vi "Shoot into low goal.vi"(6 "navX Device":T1 {"Interface"."Update Rate (4Hz-60Hz)" min=4 max=60 step=1}, 8 "Enum":enum16{"5", "4", "3", "2", "1"}(ring), 9 "SonarMB1010AnalogDevRef":T11 {"Average Bits" max=15}, 10 "MotorControlDevRef":T4, 11 "RobotDriveDevRef":T3) -> ()   [LabVIEW 2015]
uses:
  <vilib>/Rock Robotics/WPI/MotorControl/WPI_MotorControlDeviceRef.ctl
  <vilib>/Rock Robotics/WPI/MotorControl/WPI_MotorControlType.ctl
  <vilib>/Rock Robotics/SystemInterfaces/DIO/FPGA_DIOPWMChannel.ctl
  <vilib>/Rock Robotics/WPI/PWM/WPI_PWMDeadband.ctl
  <vilib>/Rock Robotics/WPI/CAN/Jaguar/SubVIs/WPI_CANJaguar_ControlMode.ctl
  <vilib>/Rock Robotics/WPI/CAN/TalonSRX/WPI_CANTalonSRX_APIControlMode.ctl
  <vilib>/Rock Robotics/WPI/Ultrasonic/WPI_SonarMB1010AnalogDeviceRef.ctl
  <vilib>/Rock Robotics/WPI/AnalogChannel/WPI_AnalogChannelDevRef.ctl
  <vilib>/Rock Robotics/SystemInterfaces/AI/FPGA_AIChannel.ctl
  <vilib>/Rock Robotics/WPI/RobotDrive/WPI_RobotDriveDevRef.ctl
  navx-mxp/labview/navX Library v2/TypeDefs/Z900_navX_DeviceTypeDef.ctl
  navx-mxp/labview/navX Library v2/TypeDefs/Z900_navX_ProtocolTypeDef.ctl
  navx-mxp/labview/navX Library v2/TypeDefs/Z900_navX_NotifyPacketTypeDef.ctl
  navx-mxp/labview/navX Library v2/TypeDefs/Z900_navX_ActionTypeDef.ctl
  <vilib>/Rock Robotics/WPI/RobotDrive/WPI_RobotDriveArcadeDrive_Standard(NoSaturation).vi
  <vilib>/Rock Robotics/WPI/Ultrasonic/WPI_SonarMB1010AnalogGetRange.vi
  navx-mxp/labview/navX Library v2/navX Library v2.lvlib
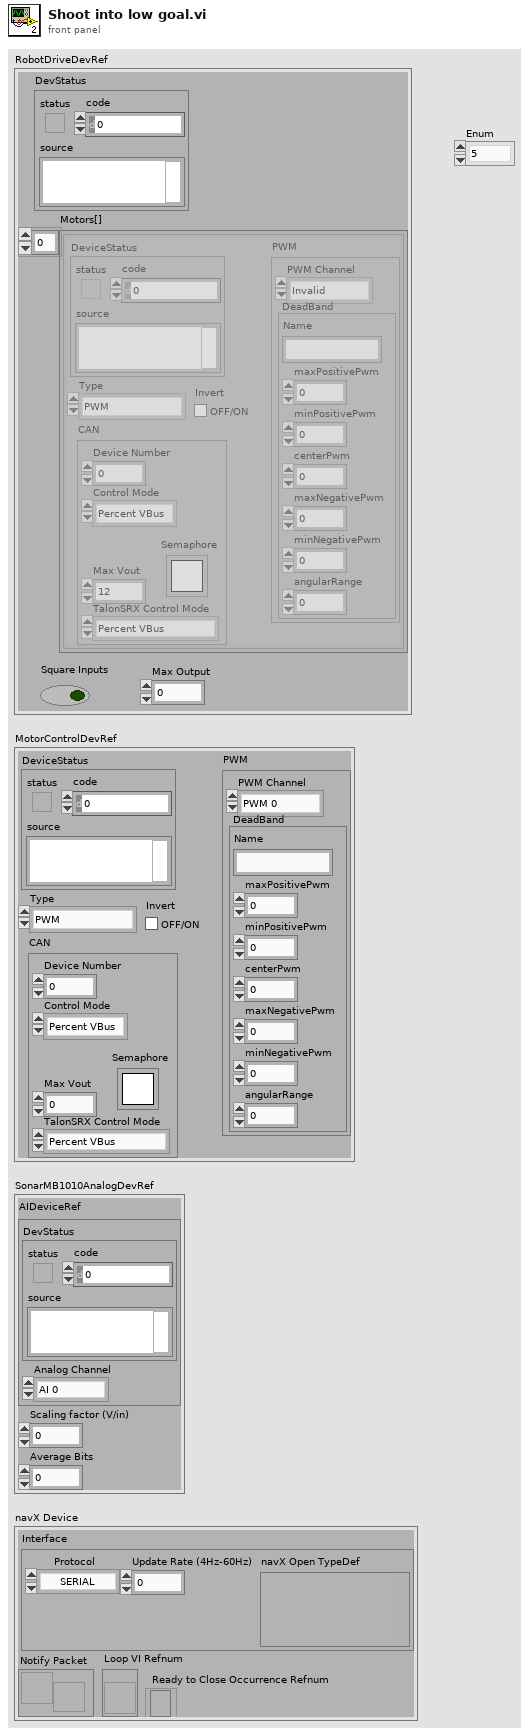
[diagram p1: front panel]
types:
  T1 = typedef "navX Library v2.lvlib/Z900_navX_DeviceTypeDef.ctl" = cluster{"Interface":cluster{"Protocol":T2, "Update Rate (4Hz-60Hz)":u8, "navX Open TypeDef":variant}, "Notify Packet":refnum<notifier>, "Loop VI Refnum":refnum<vi>, "Ready to Close Occurrence Refnum":refnum<k4>}
  T2 = typedef "navX Library v2.lvlib/Z900_navX_ProtocolTypeDef.ctl" = enum16{"SERIAL", "I2C", "SPI"}
  T3 = typedef "WPI_RobotDriveDevRef.ctl" = cluster{"DevStatus":errorcluster, "Motors[]":T4[], "Square Inputs":bool, "Max Output":dbl}
  T4 = typedef "WPI_MotorControlDeviceRef.ctl" = cluster{"DeviceStatus":errorcluster, "Type":T5, "PWM":cluster{"PWM Channel":T6, "DeadBand":T7}, "CAN":cluster{"Device Number":u8, "Control Mode":T8, "Semaphore":T9, "Max Vout":dbl, "TalonSRX Control Mode":T10}, "Invert":bool}
  T5 = typedef "WPI_MotorControlType.ctl" = enum16{"PWM", "CAN", "CANTalonSRX"}
  T6 = typedef "FPGA_DIOPWMChannel.ctl" = enum8{"PWM 0", "PWM 1", "PWM 2", "PWM 3", "PWM 4", "PWM 5", "PWM 6", "PWM 7", "PWM 8", "PWM 9", "PWM MXP 0", "PWM MXP 1", "PWM MXP 2", "PWM MXP 3", "PWM MXP 4", "PWM MXP 5", "PWM MXP 6", "PWM MXP 7", "PWM MXP 8", "PWM MXP 9", "Invalid"}
  T7 = typedef "WPI_PWMDeadband.ctl" = cluster{"Name":string, "maxPositivePwm":i32, "minPositivePwm":i32, "centerPwm":i32, "maxNegativePwm":i32, "minNegativePwm":i32, "angularRange":u16}
  T8 = typedef "WPI_CANJaguar_ControlMode.ctl" = enum8{"Percent VBus", "Current", "Speed", "Position", "Voltage"}
  T9 = typedef "Semaphore RefNum" = refnum<k1>
  T10 = typedef "WPI_CANTalonSRX_APIControlMode.ctl" = enum8{"Percent VBus", "Speed", "Position", "Slave", "Unchanged / Invalid", "Voltage Compensation", "Current", "Motion Profile"}
  T11 = typedef "WPI_SonarMB1010AnalogDeviceRef.ctl" = cluster{"AIDeviceRef":T12, "Scaling factor (V/in)":dbl, "Average Bits":u8}
  T12 = typedef "WPI_AnalogChannelDevRef.ctl" = cluster{"DevStatus":errorcluster, "Analog Channel":T13}
  T13 = typedef "FPGA_AIChannel.ctl" = enum8{"AI 0", "AI 1", "AI 2", "AI 3", "AI MXP 0", "AI MXP 1", "AI MXP 2", "AI MXP 3", "Invalid"}
  T14 = cluster{"Yaw":dbl, "Roll":dbl, "Pitch":dbl, "Heading":dbl, "Fused Heading":dbl}
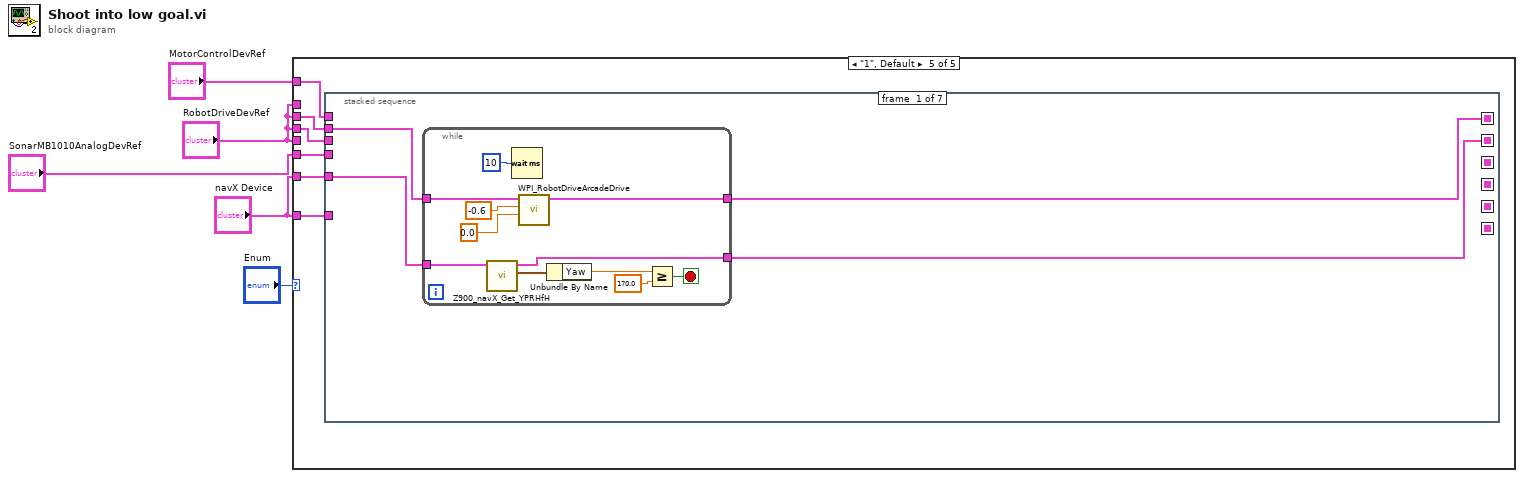
[diagram p0: block diagram]
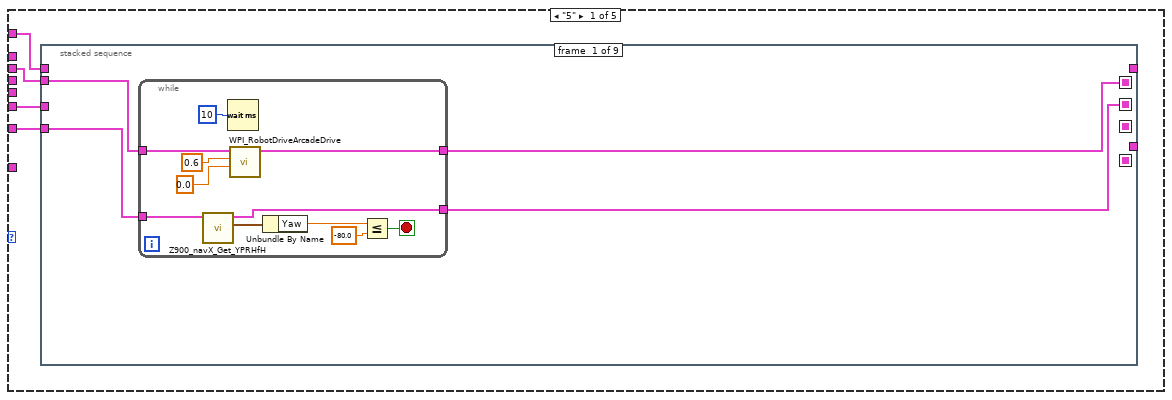
[diagram p2: hidden frame]
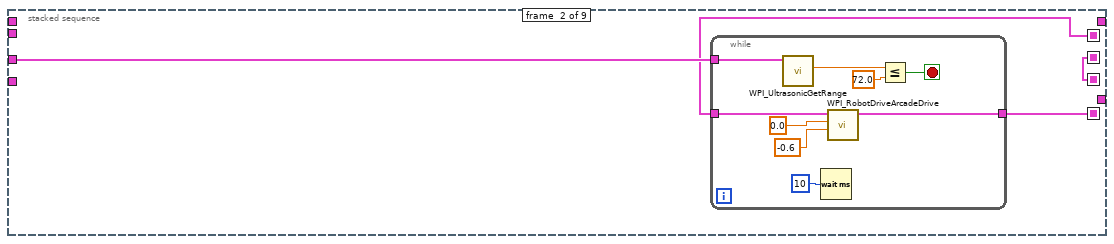
[diagram p3: hidden frame]
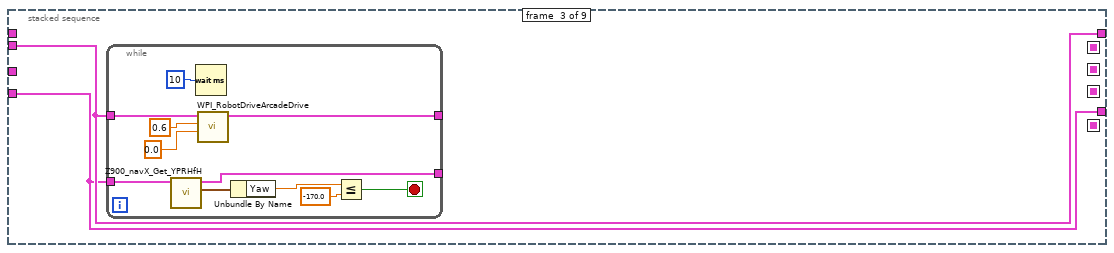
[diagram p4: hidden frame]
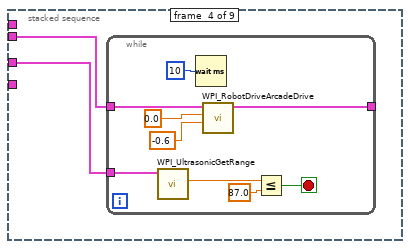
[diagram p5: hidden frame]
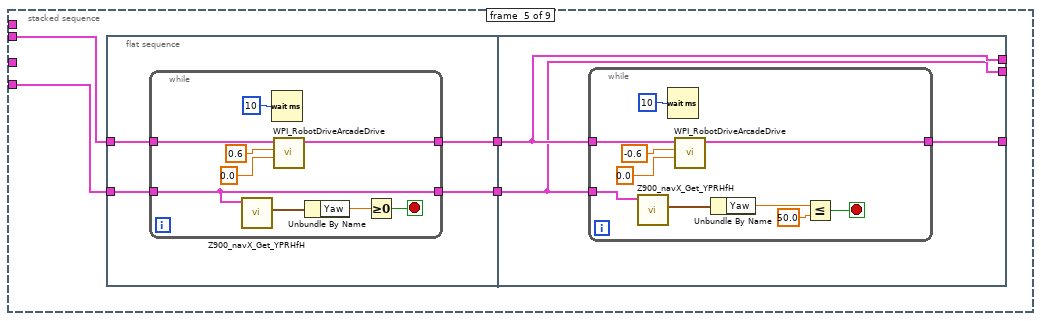
[diagram p6: hidden frame]
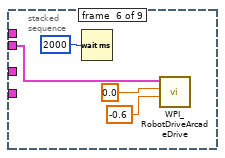
[diagram p7: hidden frame]
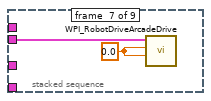
[diagram p8: hidden frame]
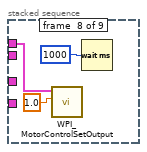
[diagram p9: hidden frame]
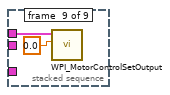
[diagram p10: hidden frame]
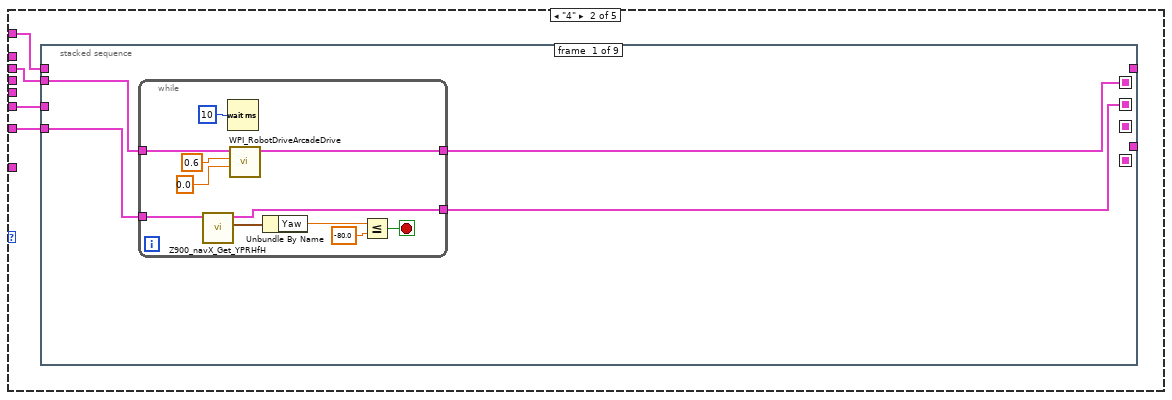
[diagram p11: hidden frame]
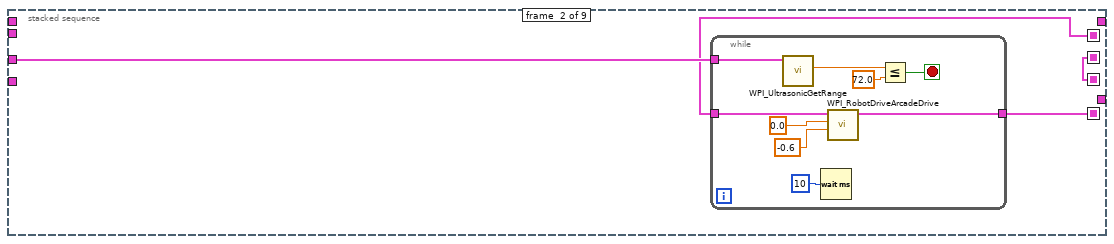
[diagram p12: hidden frame]
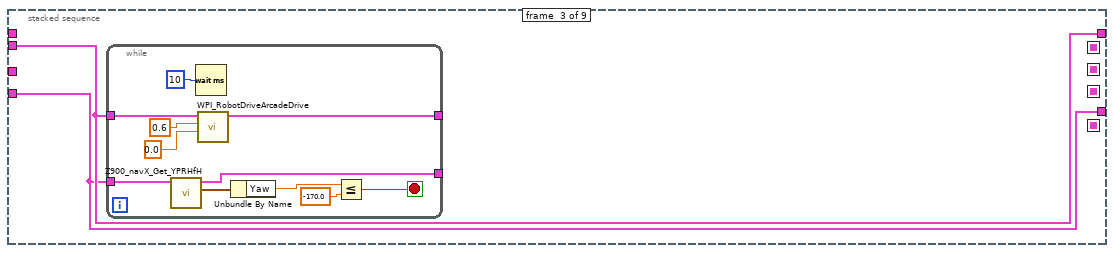
[diagram p13: hidden frame]
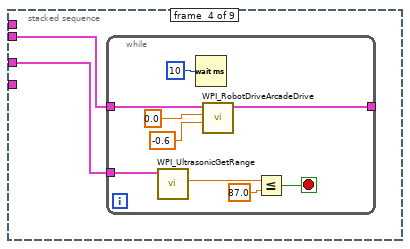
[diagram p14: hidden frame]
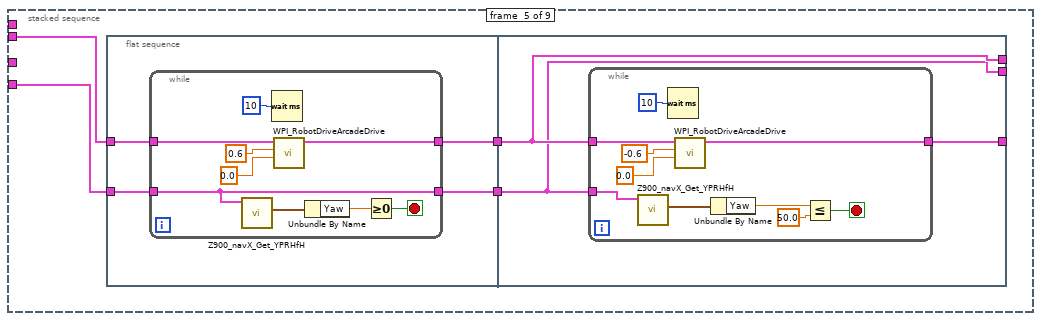
[diagram p15: hidden frame]
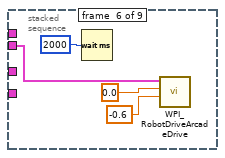
[diagram p16: hidden frame]
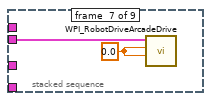
[diagram p17: hidden frame]
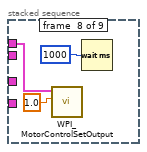
[diagram p18: hidden frame]
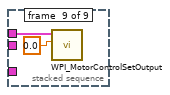
[diagram p19: hidden frame]
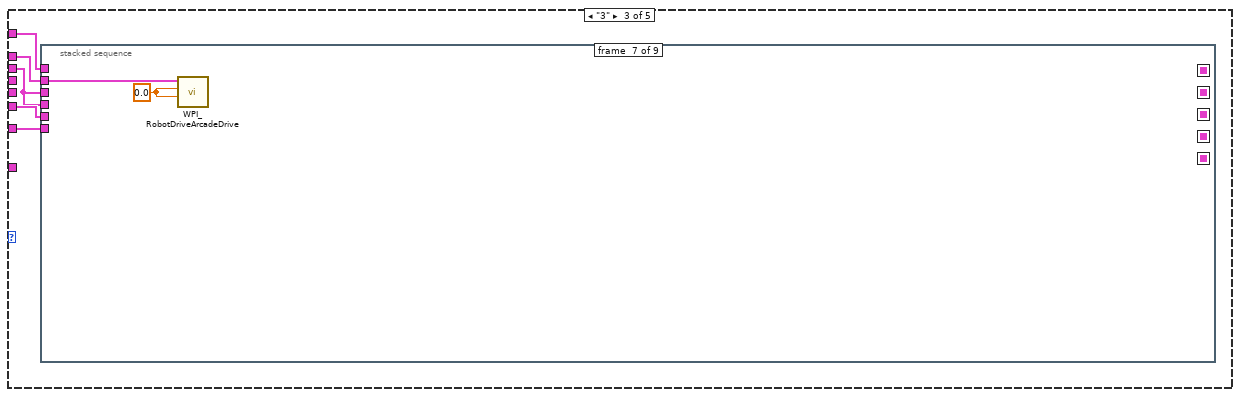
[diagram p20: hidden frame]
diagram:
  n1 = case shown="\"1\", Default" "Enum" {
    tunnel: "MotorControlDevRef" -> [w6 w103 w203 w301 w377]
    tunnel: "SonarMB1010AnalogDevRef" -> [w7 w104 w202 w300 w376]
    tunnel: "RobotDriveDevRef" -> [w9 w106 w200 w299 w375]
    tunnel: "navX Device" -> [w8 w105 w204 w298 w374]
    tunnel: "RobotDriveDevRef" -> [_ _ w201 _ _]
    tunnel: "navX Device" -> [_ _ _ _ w373]
    tunnel: "RobotDriveDevRef" -> [_ _ _ _ _]
    tunnel: "RobotDriveDevRef" -> [_ _ _ _ w372]
    frame "5" {
      n2 = stacked-sequence {
        seq-local: [w11 _ _ _ _ _ _ _ _] -> [_ w27 _ _ _ _ _ _ _]
        seq-local: [w10 _ _ _ _ _ _ _ _] -> [_ w25 _ _ _ _ _ _ _]
        seq-local: [_ w26 _ _ _ _ _ _ _] -> [_ _ _ _ _ _ _ _ _]
        seq-local: [_ w25 _ _ _ _ _ _ _] -> [_ _ _ _ _ _ _ _ _]
        tunnel: w8 -> [w12 _ w38 _ w64 _ _ _ _]
        tunnel: w9 -> [w13 _ w39 w51 w65 w92 w96 _ _]
        tunnel: w7 -> [_ w28 _ w52 _ _ _ _ _]
        tunnel: w6 -> [_ _ _ _ _ _ _ w100 w101]
        tunnel: [_ _ w38 _ _ _ _ _ _] -> _
        tunnel: [_ _ w39 _ _ _ _ _ _] -> _
        frame #0 {
          n3 = while {
            tunnel: [w21] -> w11
            tunnel: [w20] -> w10
            tunnel: w12 -> [w19]
            tunnel: w13 -> [w18]
            stop <- w15 stop-if-true
            n4 = call "Z900_navX_Get_YPRHfH.vi"("navX Device"=w19) -> ("YRPHfH"=w24:T14, "navX Device"=w20:T1)  [unwired: 7 in, 2 out]
            n5 = Wait (ms)(milliseconds to wait=u32 10) -> ()  [unwired: 1 out]
            n6 = call-poly <vilib>:"WPI_RobotDriveArcadeDrive.vi"("Y axis value"=0.0, "X axis value"=0.6, "RobotDriveDevRef"=w18) -> ("RobotDriveDevRef"=w21:T3)  [unwired: 6 in, 2 out]
            n7 = Unbundle By Name(w24) -> ("Yaw"=w17:dbl)
            n8 = Less Or Equal?(x=w17, y=-80.0) -> (x <= y?=w15:bool)
          }
        }
        frame #1 {
          n9 = while {
            tunnel: w28 -> [w37]
            tunnel: w27 -> [w31]
            tunnel: [w29] -> w26
            stop <- w34 stop-if-true
            n10 = call-poly <vilib>:"WPI_UltrasonicGetRange.vi"("SonarMB1010AnalogDevRef"=w37) -> ("Distance"=w36:dbl)  [unwired: 8 in, 2 out]
            n11 = Wait (ms)(milliseconds to wait=u32 10) -> ()  [unwired: 1 out]
            n12 = call-poly <vilib>:"WPI_RobotDriveArcadeDrive.vi"("Y axis value"=-0.6, "X axis value"=0.0, "RobotDriveDevRef"=w31) -> ("RobotDriveDevRef"=w29:T3)  [unwired: 6 in, 2 out]
            n13 = Less Or Equal?(x=w36, y=72.0) -> (x <= y?=w34:bool)
          }
        }
        frame #2 {
          n14 = while {
            tunnel: [w47] -> _
            tunnel: [w46] -> _
            tunnel: w38 -> [w45]
            tunnel: w39 -> [w44]
            stop <- w41 stop-if-true
            n15 = call "Z900_navX_Get_YPRHfH.vi"("navX Device"=w45) -> ("YRPHfH"=w50:T14, "navX Device"=w46:T1)  [unwired: 7 in, 2 out]
            n16 = Wait (ms)(milliseconds to wait=u32 10) -> ()  [unwired: 1 out]
            n17 = call-poly <vilib>:"WPI_RobotDriveArcadeDrive.vi"("Y axis value"=0.0, "X axis value"=0.6, "RobotDriveDevRef"=w44) -> ("RobotDriveDevRef"=w47:T3)  [unwired: 6 in, 2 out]
            n18 = Unbundle By Name(w50) -> ("Yaw"=w43:dbl)
            n19 = Less Or Equal?(x=w43, y=-170.0) -> (x <= y?=w41:bool)
          }
        }
        frame #3 {
          n20 = while {
            tunnel: w52 -> [w61]
            tunnel: w51 -> [w55]
            tunnel: [w53] -> _
            stop <- w58 stop-if-true
            n21 = call-poly <vilib>:"WPI_UltrasonicGetRange.vi"("SonarMB1010AnalogDevRef"=w61) -> ("Distance"=w60:dbl)  [unwired: 8 in, 2 out]
            n22 = Wait (ms)(milliseconds to wait=u32 10) -> ()  [unwired: 1 out]
            n23 = call-poly <vilib>:"WPI_RobotDriveArcadeDrive.vi"("Y axis value"=-0.6, "X axis value"=0.0, "RobotDriveDevRef"=w55) -> ("RobotDriveDevRef"=w53:T3)  [unwired: 6 in, 2 out]
            n24 = Less Or Equal?(x=w60, y=87.0) -> (x <= y?=w58:bool)
          }
        }
        frame #4 {
          n25 = flat-sequence {
            tunnel: w64 -> [w69]
            tunnel: w65 -> [w68]
            tunnel: [w67] -> w63
            tunnel: [w66] -> w62
            tunnel: [w80] -> _
            tunnel: [w79] -> _
            tunnel: [w81] -> _
            tunnel: w63 -> [w80]
            tunnel: w62 -> [w79]
            frame #0 {
              n26 = while {
                tunnel: w68 -> [w76]
                tunnel: w69 -> [w70]
                tunnel: [w72] -> w67
                tunnel: [w70] -> w66
                stop <- w77 stop-if-true
                n27 = call "Z900_navX_Get_YPRHfH.vi"("navX Device"=w70) -> ("YRPHfH"=w78:T14)  [unwired: 7 in, 3 out]
                n28 = Wait (ms)(milliseconds to wait=u32 10) -> ()  [unwired: 1 out]
                n29 = call-poly <vilib>:"WPI_RobotDriveArcadeDrive.vi"("Y axis value"=0.0, "X axis value"=0.6, "RobotDriveDevRef"=w76) -> ("RobotDriveDevRef"=w72:T3)  [unwired: 6 in, 2 out]
                n30 = Unbundle By Name(w78) -> ("Yaw"=w71:dbl)
                n31 = Greater Or Equal To 0?(x=w71) -> (x >= 0?=w77:bool)
              }
            }
            frame #1 {
              n32 = while {
                tunnel: w80 -> [w87]
                tunnel: w79 -> [w83]
                tunnel: [w82] -> w81
                stop <- w88 stop-if-true
                n33 = call "Z900_navX_Get_YPRHfH.vi"("navX Device"=w83) -> ("YRPHfH"=w91:T14)  [unwired: 7 in, 3 out]
                n34 = Wait (ms)(milliseconds to wait=u32 10) -> ()  [unwired: 1 out]
                n35 = call-poly <vilib>:"WPI_RobotDriveArcadeDrive.vi"("Y axis value"=0.0, "X axis value"=-0.6, "RobotDriveDevRef"=w87) -> ("RobotDriveDevRef"=w82:T3)  [unwired: 6 in, 2 out]
                n36 = Unbundle By Name(w91) -> ("Yaw"=w90:dbl)
                n37 = Less Or Equal?(x=w90, y=50.0) -> (x <= y?=w88:bool)
              }
            }
          }
        }
        frame #5 {
          n38 = Wait (ms)(milliseconds to wait=u32 2000) -> ()  [unwired: 1 out]
          n39 = call-poly <vilib>:"WPI_RobotDriveArcadeDrive.vi"("Y axis value"=-0.6, "X axis value"=0.0, "RobotDriveDevRef"=w92) -> ()  [unwired: 6 in, 3 out]
        }
        frame #6 {
          w97 = 0.0 ("X axis value")
          n40 = call-poly <vilib>:"WPI_RobotDriveArcadeDrive.vi"("Y axis value"=w97, "X axis value"=w97, "RobotDriveDevRef"=w96) -> ()  [unwired: 6 in, 3 out]
        }
        frame #7 {
          n41 = call <vilib>:"WPI_MotorControlSetOutput.vi"("Output"=1.0 ("Motor Output"), "MotorControlDevRef"=w100) -> ()  [unwired: 7 in, 3 out]
          n42 = Wait (ms)(milliseconds to wait=u32 1000) -> ()  [unwired: 1 out]
        }
        frame #8 {
          n43 = call <vilib>:"WPI_MotorControlSetOutput.vi"("Output"=0.0 ("Motor Output"), "MotorControlDevRef"=w101) -> ()  [unwired: 7 in, 3 out]
        }
      }
    }
    frame "4" {
      n44 = stacked-sequence {
        seq-local: [w108 _ _ _ _ _ _ _ _] -> [_ w124 _ _ _ _ _ _ _]
        seq-local: [w107 _ _ _ _ _ _ _ _] -> [_ w122 _ _ _ _ _ _ _]
        seq-local: [_ w123 _ _ _ _ _ _ _] -> [_ _ _ _ _ _ _ _ _]
        seq-local: [_ w122 _ _ _ _ _ _ _] -> [_ _ _ _ _ _ _ _ _]
        tunnel: w105 -> [w109 _ w135 _ w161 _ _ _ _]
        tunnel: w106 -> [w110 _ w136 w148 w162 w189 w193 _ _]
        tunnel: w104 -> [_ w125 _ w149 _ _ _ _ _]
        tunnel: w103 -> [_ _ _ _ _ _ _ w197 w198]
        tunnel: [_ _ w135 _ _ _ _ _ _] -> _
        tunnel: [_ _ w136 _ _ _ _ _ _] -> _
        frame #0 {
          n45 = while {
            tunnel: [w118] -> w108
            tunnel: [w117] -> w107
            tunnel: w109 -> [w116]
            tunnel: w110 -> [w115]
            stop <- w112 stop-if-true
            n46 = call "Z900_navX_Get_YPRHfH.vi"("navX Device"=w116) -> ("YRPHfH"=w121:T14, "navX Device"=w117:T1)  [unwired: 7 in, 2 out]
            n47 = Wait (ms)(milliseconds to wait=u32 10) -> ()  [unwired: 1 out]
            n48 = call-poly <vilib>:"WPI_RobotDriveArcadeDrive.vi"("Y axis value"=0.0, "X axis value"=0.6, "RobotDriveDevRef"=w115) -> ("RobotDriveDevRef"=w118:T3)  [unwired: 6 in, 2 out]
            n49 = Unbundle By Name(w121) -> ("Yaw"=w114:dbl)
            n50 = Less Or Equal?(x=w114, y=-80.0) -> (x <= y?=w112:bool)
          }
        }
        frame #1 {
          n51 = while {
            tunnel: w125 -> [w134]
            tunnel: w124 -> [w128]
            tunnel: [w126] -> w123
            stop <- w131 stop-if-true
            n52 = call-poly <vilib>:"WPI_UltrasonicGetRange.vi"("SonarMB1010AnalogDevRef"=w134) -> ("Distance"=w133:dbl)  [unwired: 8 in, 2 out]
            n53 = Wait (ms)(milliseconds to wait=u32 10) -> ()  [unwired: 1 out]
            n54 = call-poly <vilib>:"WPI_RobotDriveArcadeDrive.vi"("Y axis value"=-0.6, "X axis value"=0.0, "RobotDriveDevRef"=w128) -> ("RobotDriveDevRef"=w126:T3)  [unwired: 6 in, 2 out]
            n55 = Less Or Equal?(x=w133, y=72.0) -> (x <= y?=w131:bool)
          }
        }
        frame #2 {
          n56 = while {
            tunnel: [w144] -> _
            tunnel: [w143] -> _
            tunnel: w135 -> [w142]
            tunnel: w136 -> [w141]
            stop <- w138 stop-if-true
            n57 = call "Z900_navX_Get_YPRHfH.vi"("navX Device"=w142) -> ("YRPHfH"=w147:T14, "navX Device"=w143:T1)  [unwired: 7 in, 2 out]
            n58 = Wait (ms)(milliseconds to wait=u32 10) -> ()  [unwired: 1 out]
            n59 = call-poly <vilib>:"WPI_RobotDriveArcadeDrive.vi"("Y axis value"=0.0, "X axis value"=0.6, "RobotDriveDevRef"=w141) -> ("RobotDriveDevRef"=w144:T3)  [unwired: 6 in, 2 out]
            n60 = Unbundle By Name(w147) -> ("Yaw"=w140:dbl)
            n61 = Less Or Equal?(x=w140, y=-170.0) -> (x <= y?=w138:bool)
          }
        }
        frame #3 {
          n62 = while {
            tunnel: w149 -> [w158]
            tunnel: w148 -> [w152]
            tunnel: [w150] -> _
            stop <- w155 stop-if-true
            n63 = call-poly <vilib>:"WPI_UltrasonicGetRange.vi"("SonarMB1010AnalogDevRef"=w158) -> ("Distance"=w157:dbl)  [unwired: 8 in, 2 out]
            n64 = Wait (ms)(milliseconds to wait=u32 10) -> ()  [unwired: 1 out]
            n65 = call-poly <vilib>:"WPI_RobotDriveArcadeDrive.vi"("Y axis value"=-0.6, "X axis value"=0.0, "RobotDriveDevRef"=w152) -> ("RobotDriveDevRef"=w150:T3)  [unwired: 6 in, 2 out]
            n66 = Less Or Equal?(x=w157, y=87.0) -> (x <= y?=w155:bool)
          }
        }
        frame #4 {
          n67 = flat-sequence {
            tunnel: w161 -> [w166]
            tunnel: w162 -> [w165]
            tunnel: [w164] -> w160
            tunnel: [w163] -> w159
            tunnel: [w177] -> _
            tunnel: [w176] -> _
            tunnel: [w178] -> _
            tunnel: w160 -> [w177]
            tunnel: w159 -> [w176]
            frame #0 {
              n68 = while {
                tunnel: w165 -> [w173]
                tunnel: w166 -> [w167]
                tunnel: [w169] -> w164
                tunnel: [w167] -> w163
                stop <- w174 stop-if-true
                n69 = call "Z900_navX_Get_YPRHfH.vi"("navX Device"=w167) -> ("YRPHfH"=w175:T14)  [unwired: 7 in, 3 out]
                n70 = Wait (ms)(milliseconds to wait=u32 10) -> ()  [unwired: 1 out]
                n71 = call-poly <vilib>:"WPI_RobotDriveArcadeDrive.vi"("Y axis value"=0.0, "X axis value"=0.6, "RobotDriveDevRef"=w173) -> ("RobotDriveDevRef"=w169:T3)  [unwired: 6 in, 2 out]
                n72 = Unbundle By Name(w175) -> ("Yaw"=w168:dbl)
                n73 = Greater Or Equal To 0?(x=w168) -> (x >= 0?=w174:bool)
              }
            }
            frame #1 {
              n74 = while {
                tunnel: w177 -> [w184]
                tunnel: w176 -> [w180]
                tunnel: [w179] -> w178
                stop <- w185 stop-if-true
                n75 = call "Z900_navX_Get_YPRHfH.vi"("navX Device"=w180) -> ("YRPHfH"=w188:T14)  [unwired: 7 in, 3 out]
                n76 = Wait (ms)(milliseconds to wait=u32 10) -> ()  [unwired: 1 out]
                n77 = call-poly <vilib>:"WPI_RobotDriveArcadeDrive.vi"("Y axis value"=0.0, "X axis value"=-0.6, "RobotDriveDevRef"=w184) -> ("RobotDriveDevRef"=w179:T3)  [unwired: 6 in, 2 out]
                n78 = Unbundle By Name(w188) -> ("Yaw"=w187:dbl)
                n79 = Less Or Equal?(x=w187, y=50.0) -> (x <= y?=w185:bool)
              }
            }
          }
        }
        frame #5 {
          n80 = Wait (ms)(milliseconds to wait=u32 2000) -> ()  [unwired: 1 out]
          n81 = call-poly <vilib>:"WPI_RobotDriveArcadeDrive.vi"("Y axis value"=-0.6, "X axis value"=0.0, "RobotDriveDevRef"=w189) -> ()  [unwired: 6 in, 3 out]
        }
        frame #6 {
          w194 = 0.0 ("X axis value")
          n82 = call-poly <vilib>:"WPI_RobotDriveArcadeDrive.vi"("Y axis value"=w194, "X axis value"=w194, "RobotDriveDevRef"=w193) -> ()  [unwired: 6 in, 3 out]
        }
        frame #7 {
          n83 = call <vilib>:"WPI_MotorControlSetOutput.vi"("Output"=1.0 ("Motor Output"), "MotorControlDevRef"=w197) -> ()  [unwired: 7 in, 3 out]
          n84 = Wait (ms)(milliseconds to wait=u32 1000) -> ()  [unwired: 1 out]
        }
        frame #8 {
          n85 = call <vilib>:"WPI_MotorControlSetOutput.vi"("Output"=0.0 ("Motor Output"), "MotorControlDevRef"=w198) -> ()  [unwired: 7 in, 3 out]
        }
      }
    }
    frame "3" {
      n86 = stacked-sequence {
        seq-local: [w208 _ _ _ _ _ _ _ _] -> [_ _ _ _ _ _ _ _ _]
        seq-local: [w207 _ _ _ _ _ _ _ _] -> [_ w222 _ _ _ _ _ _ _]
        seq-local: [_ w223 _ _ _ _ _ _ _] -> [_ _ w235 _ _ _ _ _ _]
        seq-local: [_ w222 _ _ _ _ _ _ _] -> [_ _ w234 _ _ _ _ _ _]
        seq-local: [_ _ w233 _ _ _ _ _ _] -> [_ _ _ _ _ _ _ _ _]
        tunnel: w200 -> [w206 _ _ w246 w260 w287 _ _ _]
        tunnel: w204 -> [w205 _ _ _ w259 _ _ _ _]
        tunnel: w203 -> [_ _ _ _ _ _ _ w293 w296]
        tunnel: w202 -> [_ w220 _ w247 _ _ _ _ _]
        tunnel: w201 -> [_ w221 _ _ _ _ w292 _ _]
        tunnel: w200 -> [_ _ _ _ _ _ _ _ _]
        frame #0 {
          n87 = while {
            tunnel: [w216] -> w208
            tunnel: [w215] -> w207
            tunnel: w205 -> [w214]
            tunnel: w206 -> [w213]
            stop <- w210 stop-if-true
            n88 = call "Z900_navX_Get_YPRHfH.vi"("navX Device"=w214) -> ("YRPHfH"=w219:T14, "navX Device"=w215:T1)  [unwired: 7 in, 2 out]
            n89 = Wait (ms)(milliseconds to wait=u32 10) -> ()  [unwired: 1 out]
            n90 = call-poly <vilib>:"WPI_RobotDriveArcadeDrive.vi"("Y axis value"=0.0, "X axis value"=-0.6, "RobotDriveDevRef"=w213) -> ("RobotDriveDevRef"=w216:T3)  [unwired: 6 in, 2 out]
            n91 = Unbundle By Name(w219) -> ("Yaw"=w212:dbl)
            n92 = Greater Or Equal?(x=w212, y=80.0) -> (x >= y?=w210:bool)
          }
        }
        frame #1 {
          n93 = while {
            tunnel: [w226] -> w223
            tunnel: w221 -> [w225]
            tunnel: w220 -> [w224]
            stop <- w230 stop-if-true
            # "?"
            n94 = call-poly <vilib>:"WPI_UltrasonicGetRange.vi"("SonarMB1010AnalogDevRef"=w224) -> ("Distance"=w232:dbl)  [unwired: 8 in, 2 out]
            n95 = Wait (ms)(milliseconds to wait=u32 10) -> ()  [unwired: 1 out]
            n96 = call-poly <vilib>:"WPI_RobotDriveArcadeDrive.vi"("Y axis value"=-0.6, "X axis value"=0.0, "RobotDriveDevRef"=w225) -> ("RobotDriveDevRef"=w226:T3)  [unwired: 6 in, 2 out]
            n97 = Less Or Equal?(x=w232, y=82.0) -> (x <= y?=w230:bool)
          }
        }
        frame #2 {
          # "right turn"
          n98 = while {
            tunnel: w235 -> [w241]
            tunnel: w234 -> [w237]
            tunnel: [w236] -> w233
            stop <- w242 stop-if-true
            n99 = call "Z900_navX_Get_YPRHfH.vi"("navX Device"=w237) -> ("YRPHfH"=w245:T14)  [unwired: 7 in, 3 out]
            n100 = Wait (ms)(milliseconds to wait=u32 10) -> ()  [unwired: 1 out]
            n101 = call-poly <vilib>:"WPI_RobotDriveArcadeDrive.vi"("Y axis value"=0.0, "X axis value"=-0.6, "RobotDriveDevRef"=w241) -> ("RobotDriveDevRef"=w236:T3)  [unwired: 6 in, 2 out]
            n102 = Unbundle By Name(w245) -> ("Yaw"=w244:dbl)
            n103 = Greater Or Equal?(x=w244, y=170.0) -> (x >= y?=w242:bool)
          }
        }
        frame #3 {
          n104 = while {
            tunnel: w247 -> [w256]
            tunnel: w246 -> [w250]
            tunnel: [w248] -> _
            stop <- w253 stop-if-true
            n105 = call-poly <vilib>:"WPI_UltrasonicGetRange.vi"("SonarMB1010AnalogDevRef"=w256) -> ("Distance"=w255:dbl)  [unwired: 8 in, 2 out]
            n106 = Wait (ms)(milliseconds to wait=u32 10) -> ()  [unwired: 1 out]
            n107 = call-poly <vilib>:"WPI_RobotDriveArcadeDrive.vi"("Y axis value"=-0.6, "X axis value"=0.0, "RobotDriveDevRef"=w250) -> ("RobotDriveDevRef"=w248:T3)  [unwired: 6 in, 2 out]
            n108 = Less Or Equal?(x=w255, y=28.0) -> (x <= y?=w253:bool)
          }
        }
        frame #4 {
          # "left turn"
          n109 = flat-sequence {
            tunnel: w259 -> [w264]
            tunnel: w260 -> [w263]
            tunnel: [w262] -> w258
            tunnel: [w261] -> w257
            tunnel: [w275] -> _
            tunnel: [w274] -> _
            tunnel: [w276] -> _
            tunnel: w258 -> [w275]
            tunnel: w257 -> [w274]
            frame #0 {
              n110 = while {
                tunnel: w263 -> [w271]
                tunnel: w264 -> [w265]
                tunnel: [w267] -> w262
                tunnel: [w265] -> w261
                stop <- w272 stop-if-true
                n111 = call "Z900_navX_Get_YPRHfH.vi"("navX Device"=w265) -> ("YRPHfH"=w273:T14)  [unwired: 7 in, 3 out]
                n112 = Wait (ms)(milliseconds to wait=u32 10) -> ()  [unwired: 1 out]
                n113 = call-poly <vilib>:"WPI_RobotDriveArcadeDrive.vi"("Y axis value"=0.0, "X axis value"=-0.6, "RobotDriveDevRef"=w271) -> ("RobotDriveDevRef"=w267:T3)  [unwired: 6 in, 2 out]
                n114 = Unbundle By Name(w273) -> ("Yaw"=w266:dbl)
                n115 = Less Or Equal To 0?(x=w266) -> (x <= 0?=w272:bool)
              }
            }
            frame #1 {
              n116 = while {
                tunnel: w275 -> [w282]
                tunnel: w274 -> [w278]
                tunnel: [w277] -> w276
                stop <- w283 stop-if-true
                n117 = call "Z900_navX_Get_YPRHfH.vi"("navX Device"=w278) -> ("YRPHfH"=w286:T14)  [unwired: 7 in, 3 out]
                n118 = Wait (ms)(milliseconds to wait=u32 10) -> ()  [unwired: 1 out]
                n119 = call-poly <vilib>:"WPI_RobotDriveArcadeDrive.vi"("Y axis value"=0.0, "X axis value"=-0.6, "RobotDriveDevRef"=w282) -> ("RobotDriveDevRef"=w277:T3)  [unwired: 6 in, 2 out]
                n120 = Unbundle By Name(w286) -> ("Yaw"=w285:dbl)
                n121 = Greater Or Equal?(x=w285, y=-130.0) -> (x >= y?=w283:bool)
              }
            }
          }
        }
        frame #5 {
          n122 = Wait (ms)(milliseconds to wait=u32 2000) -> ()  [unwired: 1 out]
          n123 = call-poly <vilib>:"WPI_RobotDriveArcadeDrive.vi"("Y axis value"=-0.6, "X axis value"=0.0, "RobotDriveDevRef"=w287) -> ()  [unwired: 6 in, 3 out]
        }
        frame #6 {
          w291 = 0.0 ("X axis value")
          n124 = call-poly <vilib>:"WPI_RobotDriveArcadeDrive.vi"("Y axis value"=w291, "X axis value"=w291, "RobotDriveDevRef"=w292) -> ()  [unwired: 6 in, 3 out]
        }
        frame #7 {
          n125 = call <vilib>:"WPI_MotorControlSetOutput.vi"("Output"=1.0 ("Motor Output"), "MotorControlDevRef"=w293) -> ()  [unwired: 7 in, 3 out]
          n126 = Wait (ms)(milliseconds to wait=u32 1000) -> ()  [unwired: 1 out]
        }
        frame #8 {
          n127 = call <vilib>:"WPI_MotorControlSetOutput.vi"("Output"=0.0, "MotorControlDevRef"=w296) -> ()  [unwired: 7 in, 3 out]
        }
      }
    }
    frame "2" {
      n128 = stacked-sequence {
        seq-local: [w303 _ _ _ _ _ _] -> [_ w319 _ _ _ _ _]
        seq-local: [w302 _ _ _ _ _ _] -> [_ w317 _ _ _ _ _]
        seq-local: [_ w318 _ _ _ _ _] -> [_ _ w334 _ _ _ _]
        seq-local: [_ w317 _ _ _ _ _] -> [_ _ w333 _ _ _ _]
        seq-local: [_ _ w332 _ _ _ _] -> [_ _ _ w363 _ _ _]
        seq-local: [_ _ _ w359 _ _ _] -> [_ _ _ _ w365 _ _]
        tunnel: w298 -> [w304 _ w330 _ _ _ _]
        tunnel: w299 -> [w305 _ w331 _ _ _ _]
        tunnel: w300 -> [_ w320 _ _ _ _ _]
        tunnel: w301 -> [_ _ _ _ _ w369 w370]
        tunnel: [_ _ w330 _ _ _ _] -> _
        tunnel: [_ _ w331 _ _ _ _] -> _
        frame #0 {
          n129 = while {
            tunnel: [w313] -> w303
            tunnel: [w312] -> w302
            tunnel: w304 -> [w311]
            tunnel: w305 -> [w310]
            stop <- w307 stop-if-true
            n130 = call "Z900_navX_Get_YPRHfH.vi"("navX Device"=w311) -> ("YRPHfH"=w316:T14, "navX Device"=w312:T1)  [unwired: 7 in, 2 out]
            n131 = Wait (ms)(milliseconds to wait=u32 10) -> ()  [unwired: 1 out]
            n132 = call-poly <vilib>:"WPI_RobotDriveArcadeDrive.vi"("Y axis value"=0.0, "X axis value"=-0.6, "RobotDriveDevRef"=w310) -> ("RobotDriveDevRef"=w313:T3)  [unwired: 6 in, 2 out]
            n133 = Unbundle By Name(w316) -> ("Yaw"=w309:dbl)
            n134 = Greater Or Equal?(x=w309, y=170.0) -> (x >= y?=w307:bool)
          }
        }
        frame #1 {
          n135 = while {
            tunnel: w320 -> [w329]
            tunnel: w319 -> [w323]
            tunnel: [w321] -> w318
            stop <- w326 stop-if-true
            n136 = call-poly <vilib>:"WPI_UltrasonicGetRange.vi"("SonarMB1010AnalogDevRef"=w329) -> ("Distance"=w328:dbl)  [unwired: 8 in, 2 out]
            n137 = Wait (ms)(milliseconds to wait=u32 10) -> ()  [unwired: 1 out]
            n138 = call-poly <vilib>:"WPI_RobotDriveArcadeDrive.vi"("Y axis value"=-0.6, "X axis value"=0.0, "RobotDriveDevRef"=w323) -> ("RobotDriveDevRef"=w321:T3)  [unwired: 6 in, 2 out]
            n139 = Less Or Equal?(x=w328, y=28.0) -> (x <= y?=w326:bool)
          }
        }
        frame #2 {
          n140 = flat-sequence {
            tunnel: w330 -> [w336]
            tunnel: w331 -> [w335]
            tunnel: w334 -> [w348]
            tunnel: w333 -> [w347]
            tunnel: [w346] -> w332
            frame #0 {
              n141 = while {
                tunnel: w335 -> [w343]
                tunnel: w336 -> [w339]
                tunnel: [w338] -> _
                stop <- w344 stop-if-true
                n142 = call "Z900_navX_Get_YPRHfH.vi"("navX Device"=w339) -> ("YRPHfH"=w345:T14)  [unwired: 7 in, 3 out]
                n143 = Wait (ms)(milliseconds to wait=u32 10) -> ()  [unwired: 1 out]
                n144 = call-poly <vilib>:"WPI_RobotDriveArcadeDrive.vi"("Y axis value"=0.0, "X axis value"=-0.6, "RobotDriveDevRef"=w343) -> ("RobotDriveDevRef"=w338:T3)  [unwired: 6 in, 2 out]
                n145 = Unbundle By Name(w345) -> ("Yaw"=w337:dbl)
                n146 = Less Or Equal To 0?(x=w337) -> (x <= 0?=w344:bool)
              }
            }
            frame #1 {
              n147 = while {
                tunnel: w348 -> [w354]
                tunnel: w347 -> [w350]
                tunnel: [w349] -> w346
                stop <- w355 stop-if-true
                n148 = call "Z900_navX_Get_YPRHfH.vi"("navX Device"=w350) -> ("YRPHfH"=w358:T14)  [unwired: 7 in, 3 out]
                n149 = Wait (ms)(milliseconds to wait=u32 10) -> ()  [unwired: 1 out]
                n150 = call-poly <vilib>:"WPI_RobotDriveArcadeDrive.vi"("Y axis value"=0.0, "X axis value"=-0.6, "RobotDriveDevRef"=w354) -> ("RobotDriveDevRef"=w349:T3)  [unwired: 6 in, 2 out]
                n151 = Unbundle By Name(w358) -> ("Yaw"=w357:dbl)
                n152 = Greater Or Equal?(x=w357, y=-130.0) -> (x >= y?=w355:bool)
              }
            }
          }
        }
        frame #3 {
          n153 = Wait (ms)(milliseconds to wait=u32 2000) -> ()  [unwired: 1 out]
          n154 = call-poly <vilib>:"WPI_RobotDriveArcadeDrive.vi"("Y axis value"=-0.6, "X axis value"=0.0, "RobotDriveDevRef"=w363) -> ("RobotDriveDevRef"=w359:T3)  [unwired: 6 in, 2 out]
        }
        frame #4 {
          n155 = call-poly <vilib>:"WPI_RobotDriveArcadeDrive.vi"("Y axis value"=0.0, "X axis value"=0.0, "RobotDriveDevRef"=w365) -> ()  [unwired: 6 in, 3 out]
        }
        frame #5 {
          n156 = call <vilib>:"WPI_MotorControlSetOutput.vi"("Output"=1.0 ("Motor Output"), "MotorControlDevRef"=w369) -> ()  [unwired: 7 in, 3 out]
          n157 = Wait (ms)(milliseconds to wait=u32 1000) -> ()  [unwired: 1 out]
        }
        frame #6 {
          n158 = call <vilib>:"WPI_MotorControlSetOutput.vi"("Output"=0.0 ("Motor Output"), "MotorControlDevRef"=w370) -> ()  [unwired: 7 in, 3 out]
        }
      }
    }
    frame "1", Default {
      n159 = stacked-sequence {
        seq-local: [w379 _ _ _ _ _ _] -> [_ w395 _ _ _ _ _]
        seq-local: [w378 _ _ _ _ _ _] -> [_ w393 _ _ _ _ _]
        seq-local: [_ w394 _ _ _ _ _] -> [_ _ w410 _ _ _ _]
        seq-local: [_ w393 _ _ _ _ _] -> [_ _ w409 _ _ _ _]
        seq-local: [_ _ w408 _ _ _ _] -> [_ _ _ w439 _ _ _]
        seq-local: [_ _ _ w435 _ _ _] -> [_ _ _ _ w441 _ _]
        tunnel: w374 -> [w380 _ _ _ _ _ _]
        tunnel: w375 -> [w381 _ _ _ _ _ _]
        tunnel: w376 -> [_ w396 _ _ _ _ _]
        tunnel: w377 -> [_ _ _ _ _ w445 w446]
        tunnel: w373 -> [_ _ w407 _ _ _ _]
        tunnel: w372 -> [_ _ w406 _ _ _ _]
        frame #0 {
          n160 = while {
            tunnel: [w389] -> w379
            tunnel: [w388] -> w378
            tunnel: w380 -> [w387]
            tunnel: w381 -> [w386]
            stop <- w383 stop-if-true
            n161 = call "Z900_navX_Get_YPRHfH.vi"("navX Device"=w387) -> ("YRPHfH"=w392:T14, "navX Device"=w388:T1)  [unwired: 7 in, 2 out]
            n162 = Wait (ms)(milliseconds to wait=u32 10) -> ()  [unwired: 1 out]
            n163 = call-poly <vilib>:"WPI_RobotDriveArcadeDrive.vi"("Y axis value"=0.0, "X axis value"=-0.6, "RobotDriveDevRef"=w386) -> ("RobotDriveDevRef"=w389:T3)  [unwired: 6 in, 2 out]
            n164 = Unbundle By Name(w392) -> ("Yaw"=w385:dbl)
            n165 = Greater Or Equal?(x=w385, y=170.0) -> (x >= y?=w383:bool)
          }
        }
        frame #1 {
          n166 = while {
            tunnel: w396 -> [w405]
            tunnel: w395 -> [w399]
            tunnel: [w397] -> w394
            stop <- w402 stop-if-true
            n167 = call-poly <vilib>:"WPI_UltrasonicGetRange.vi"("SonarMB1010AnalogDevRef"=w405) -> ("Distance"=w404:dbl)  [unwired: 8 in, 2 out]
            n168 = Wait (ms)(milliseconds to wait=u32 10) -> ()  [unwired: 1 out]
            n169 = call-poly <vilib>:"WPI_RobotDriveArcadeDrive.vi"("Y axis value"=-0.6, "X axis value"=0.0, "RobotDriveDevRef"=w399) -> ("RobotDriveDevRef"=w397:T3)  [unwired: 6 in, 2 out]
            n170 = Less Or Equal?(x=w404, y=44.0) -> (x <= y?=w402:bool)
          }
        }
        frame #2 {
          n171 = flat-sequence {
            tunnel: w407 -> [w412]
            tunnel: w406 -> [w411]
            tunnel: w410 -> [w424]
            tunnel: w409 -> [w423]
            tunnel: [w422] -> w408
            frame #0 {
              n172 = while {
                tunnel: w411 -> [w419]
                tunnel: w412 -> [w415]
                tunnel: [w414] -> _
                stop <- w420 stop-if-true
                n173 = call "Z900_navX_Get_YPRHfH.vi"("navX Device"=w415) -> ("YRPHfH"=w421:T14)  [unwired: 7 in, 3 out]
                n174 = Wait (ms)(milliseconds to wait=u32 10) -> ()  [unwired: 1 out]
                n175 = call-poly <vilib>:"WPI_RobotDriveArcadeDrive.vi"("Y axis value"=0.0, "X axis value"=-0.6, "RobotDriveDevRef"=w419) -> ("RobotDriveDevRef"=w414:T3)  [unwired: 6 in, 2 out]
                n176 = Unbundle By Name(w421) -> ("Yaw"=w413:dbl)
                n177 = Less Or Equal To 0?(x=w413) -> (x <= 0?=w420:bool)
              }
            }
            frame #1 {
              n178 = while {
                tunnel: w424 -> [w430]
                tunnel: w423 -> [w426]
                tunnel: [w425] -> w422
                stop <- w431 stop-if-true
                n179 = call "Z900_navX_Get_YPRHfH.vi"("navX Device"=w426) -> ("YRPHfH"=w434:T14)  [unwired: 7 in, 3 out]
                n180 = Wait (ms)(milliseconds to wait=u32 10) -> ()  [unwired: 1 out]
                n181 = call-poly <vilib>:"WPI_RobotDriveArcadeDrive.vi"("Y axis value"=0.0, "X axis value"=-0.6, "RobotDriveDevRef"=w430) -> ("RobotDriveDevRef"=w425:T3)  [unwired: 6 in, 2 out]
                n182 = Unbundle By Name(w434) -> ("Yaw"=w433:dbl)
                n183 = Greater Or Equal?(x=w433, y=-130.0) -> (x >= y?=w431:bool)
              }
            }
          }
        }
        frame #3 {
          n184 = Wait (ms)(milliseconds to wait=u32 4000) -> ()  [unwired: 1 out]
          n185 = call-poly <vilib>:"WPI_RobotDriveArcadeDrive.vi"("Y axis value"=-0.6, "X axis value"=0.0, "RobotDriveDevRef"=w439) -> ("RobotDriveDevRef"=w435:T3)  [unwired: 6 in, 2 out]
        }
        frame #4 {
          n186 = call-poly <vilib>:"WPI_RobotDriveArcadeDrive.vi"("Y axis value"=0.0, "X axis value"=0.0, "RobotDriveDevRef"=w441) -> ()  [unwired: 6 in, 3 out]
        }
        frame #5 {
          n187 = call <vilib>:"WPI_MotorControlSetOutput.vi"("Output"=1.0 ("Motor Output"), "MotorControlDevRef"=w445) -> ()  [unwired: 7 in, 3 out]
          n188 = Wait (ms)(milliseconds to wait=u32 1000) -> ()  [unwired: 1 out]
        }
        frame #6 {
          n189 = call <vilib>:"WPI_MotorControlSetOutput.vi"("Output"=0.0 ("Motor Output"), "MotorControlDevRef"=w446) -> ()  [unwired: 7 in, 3 out]
        }
      }
    }
  }
